vi "AUTON_Index.vi"(0 "Auton Array":dbl[][](array[numeric]), 5 "MeasuredHeading":dbl, 7 "LeftEncoder":dbl, 9 "RightEncoder":dbl) -> (4 "Left Drive":dbl, 6 "Right Drive":dbl)   [LabVIEW 2012]
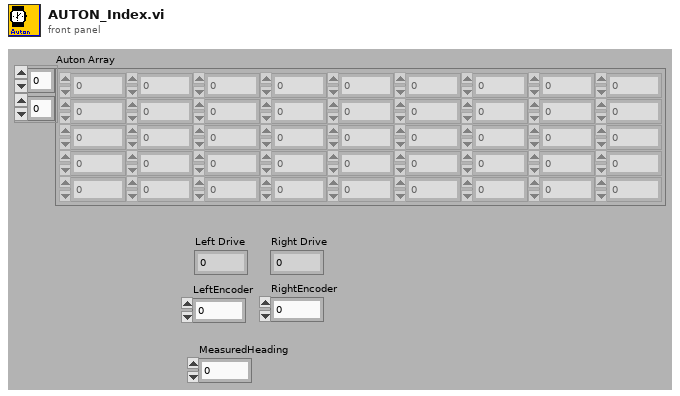
[diagram p1: front panel]
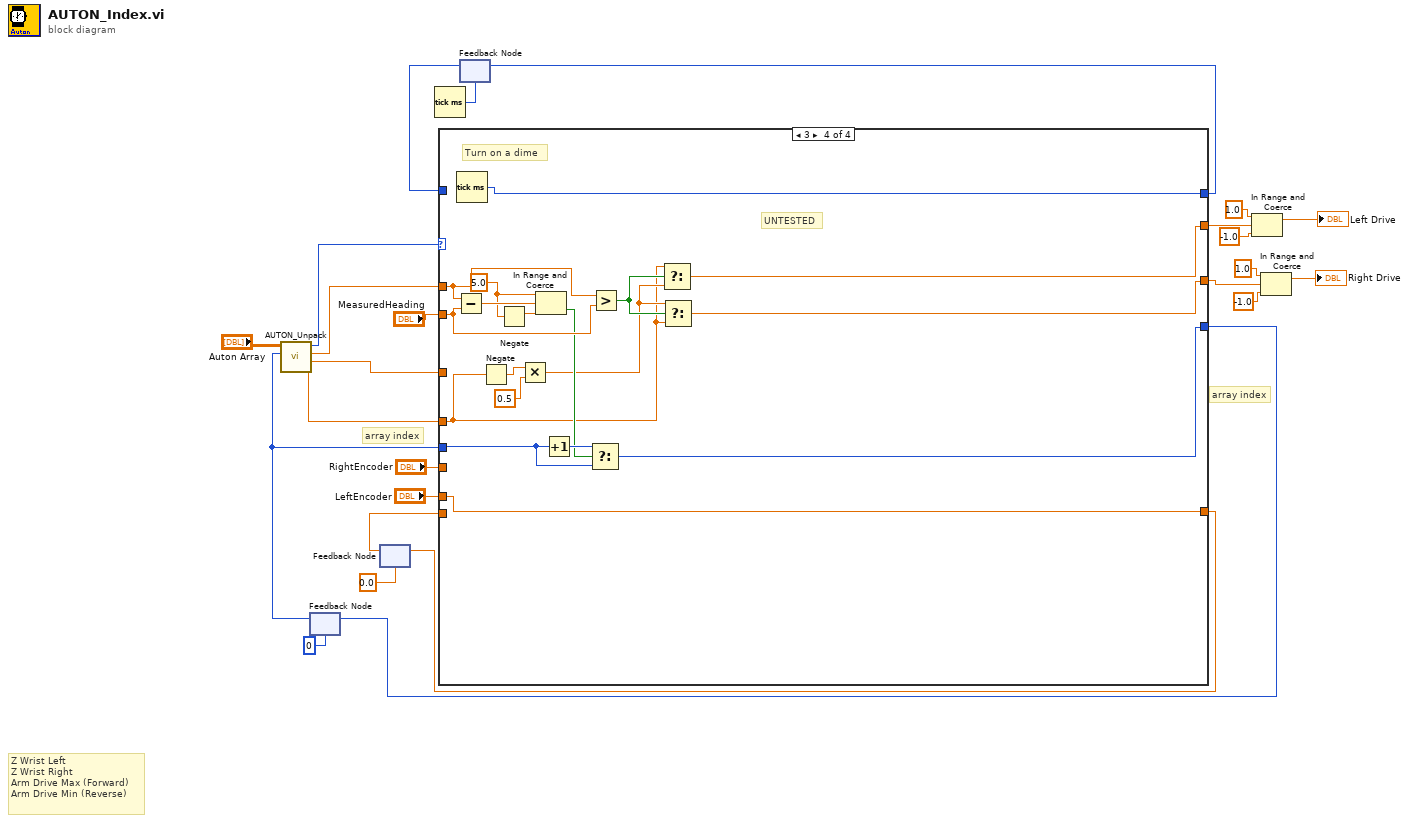
[diagram p0: block diagram]
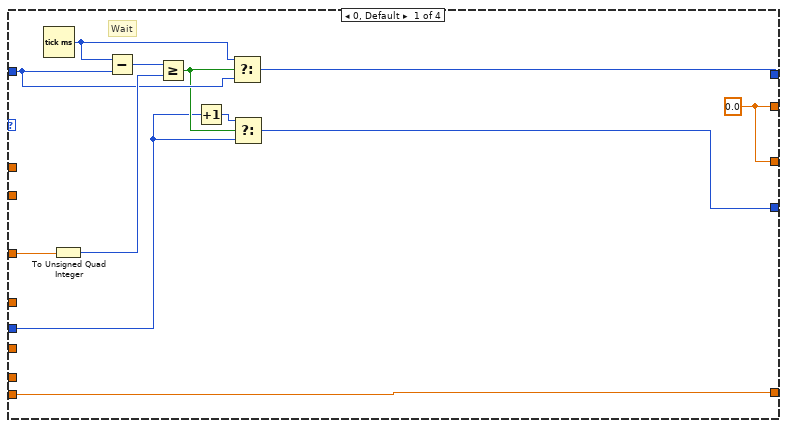
[diagram p2: hidden frame]
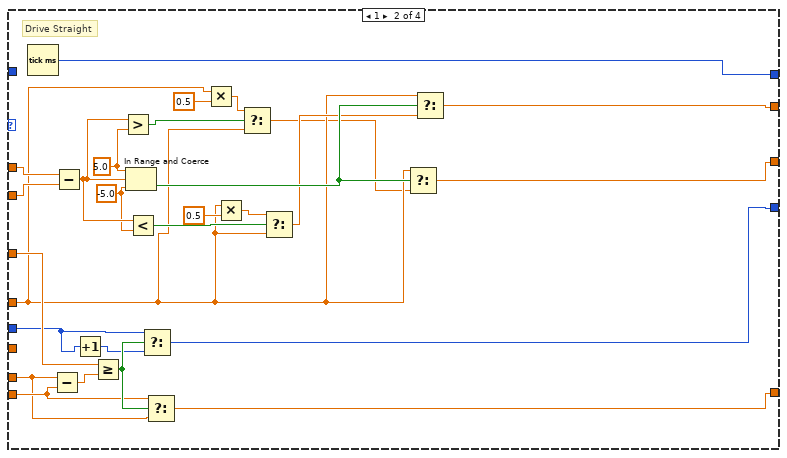
[diagram p3: hidden frame]
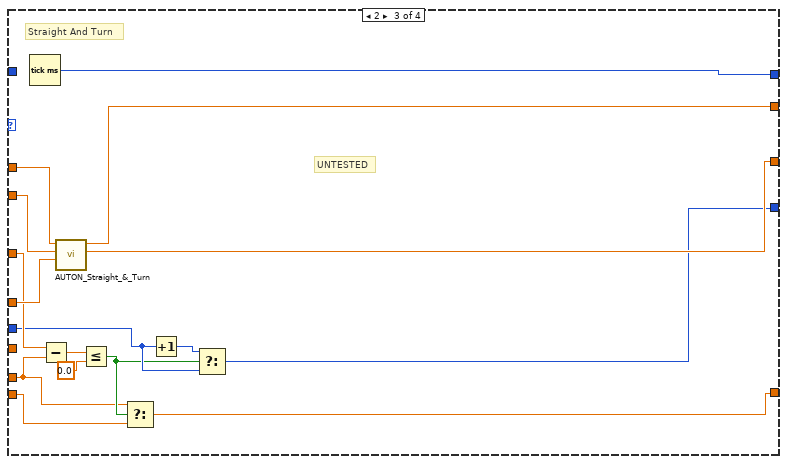
[diagram p4: hidden frame]
diagram:
  # "Z Wrist Left\nZ Wrist Right\nArm Drive Max (Forward)\nArm Drive Min (Reverse)"
  # "array index"
  # "array index"
  n1 = feedback #1(0) -> (w1:i32)
  n2 = call "AUTON_Unpack.vi"("Index"=w1, "all rows"="Auton Array") -> ("Power"=w4:dbl, "Time/Distance"=w2:dbl, "Desired Heading"=w3:dbl, "Primitive ID"=w5:i16)  [unwired: 4 in, 2 out]
  n3 = feedback #2(0.0) -> (w7:dbl)
  n4 = Tick Count (ms)() -> (millisecond timer value=w22:u32)
  n5 = feedback #3(w22) -> (w24:u32)
  n6 = case shown="3" w5 {
    tunnel: [w29 w60 w69 w93] -> w10
    tunnel: w1 -> [w30 w41 w70 w96]
    tunnel: [w37 w38 w75 w98] -> w12
    tunnel: w24 -> [w34 _ _ _]
    tunnel: w2 -> [w27 w62 w74 _]
    tunnel: w3 -> [_ w59 w80 w88]
    tunnel: [w28 w56 w77 w94] -> w20
    tunnel: [w28 w55 w76 w95] -> w13
    tunnel: w4 -> [_ w44 w78 w81]
    tunnel: "LeftEncoder" -> [_ w39 w66 w92]
    tunnel: "MeasuredHeading" -> [_ w58 w79 w87]
    tunnel: "RightEncoder" -> [_ _ _ _]
    tunnel: w7 -> [w26 w40 w67 _]
    tunnel: [w26 w64 w65 w92] -> w6
    frame 0, Default {
      w28 = 0.0 ("Numeric")
      # "Wait"
      n7 = Tick Count (ms)() -> (millisecond timer value=w33:u32)
      n8 = To Unsigned Quad Integer(1:w27) -> (0:w35:u64)
      n9 = Subtract(x=w33, y=w34) -> (x-y=w36:u32)
      n10 = Greater Or Equal?(x=w36, y=w35) -> (x >= y?=w32:bool)
      n11 = Increment(x=w30) -> (x+1=w31:i32)
      n12 = Select(t=w33, s=w32, f=w34) -> (s? t:f=w37:u32)
      n13 = Select(t=w31, s=w32, f=w30) -> (s? t:f=w29:i32)
    }
    frame 1 {
      w52 = -5.0 ("lower limit")
      w54 = 5.0 ("upper limit")
      # "Drive Straight"
      n14 = Tick Count (ms)() -> (millisecond timer value=w38:u32)
      n15 = Subtract(x=w39, y=w40) -> (x-y=w63:dbl)
      n16 = Subtract(x=w59, y=w58) -> (x-y=w53:dbl)
      n17 = Increment(x=w41) -> (x+1=w42:i32)
      n18 = Greater Or Equal?(x=w62, y=w63) -> (x >= y?=w61:bool)
      n19 = Greater?(x=w53, y=w54) -> (0:w47:bool)
      n20 = In Range and Coerce(upper limit=w54, x=w53, lower limit=w52) -> (In Range?=w57:bool)  [unwired: 1 out]
      n21 = Less?(x=w53, y=w52) -> (x < y?=w51:bool)
      n22 = Select(t=w41, s=w61, f=w42) -> (s? t:f=w60:i32)
      n23 = Select(t=w40, s=w61, f=w39) -> (s? t:f=w64:dbl)
      n24 = Multiply(x=w44, y=0.5) -> (x*y=w46:dbl)
      n25 = Multiply(x=w44, y=0.5) -> (x*y=w49:dbl)
      n26 = Select(t=w46, s=w47, f=w44) -> (s? t:f=w43:dbl)
      n27 = Select(t=w49, s=w51, f=w44) -> (s? t:f=w48:dbl)
      n28 = Select(t=w44, s=w57, f=w43) -> (s? t:f=w55:dbl)
      n29 = Select(t=w44, s=w57, f=w48) -> (s? t:f=w56:dbl)
    }
    frame 2 {
      # "UNTESTED"
      # "Straight And Turn"
      n30 = Tick Count (ms)() -> (millisecond timer value=w75:u32)
      n31 = Subtract(x=w74, y=w66) -> (x-y=w73:dbl)
      n32 = call "AUTON_Straight_&_Turn.vi"("Power"=w78, "Current Heading"=w79, "Desired Heading"=w80) -> ("Right Drive"=w76:dbl, "Left Drive"=w77:dbl)  [unwired: 7 in]
      n33 = Less Or Equal?(x=w73, y=0.0) -> (x <= y?=w68:bool)
      n34 = Select(t=w66, s=w68, f=w67) -> (s? t:f=w65:dbl)
      n35 = Increment(x=w70) -> (x+1=w71:i32)
      n36 = Select(t=w71, s=w68, f=w70) -> (s? t:f=w69:i32)
    }
    frame 3 {
      w89 = 5.0 ("upper limit")
      # "UNTESTED"
      # "Turn on a dime"
      n37 = Subtract(x=w88, y=w87) -> (x-y=w91:dbl)
      n38 = Tick Count (ms)() -> (millisecond timer value=w98:u32)
      n39 = Negate(x=w81) -> (-x=w84:dbl)
      n40 = Negate(x=w89) -> (-x=w90:dbl)
      n41 = Multiply(x=w84, y=0.5) -> (x*y=w82:dbl)
      n42 = In Range and Coerce(upper limit=w89, x=w91, lower limit=w90) -> (In Range?=w86:bool)  [unwired: 1 out]
      n43 = Increment(x=w96) -> (x+1=w97:i32)
      n44 = Select(t=w97, s=w86, f=w96) -> (s? t:f=w93:i32)
      n45 = Greater?(x=w88, y=w87) -> (0:w85:bool)
      n46 = Select(t=w81, s=w85, f=w82) -> (s? t:f=w94:dbl)
      n47 = Select(t=w82, s=w85, f=w81) -> (s? t:f=w95:dbl)
    }
  }
  n48 = feedback-in #1(w10) -> ()
  n49 = feedback-in #2(w6) -> ()
  n50 = feedback-in #3(w12) -> ()
  n51 = In Range and Coerce(upper limit=1.0, x=w20, lower limit=-1.0) -> (coerced(x)=→"Left Drive":dbl)  [unwired: 1 out]
  n52 = In Range and Coerce(upper limit=1.0, x=w13, lower limit=-1.0) -> (coerced(x)=→"Right Drive":dbl)  [unwired: 1 out]
